vi "ConvertTextBasedCodeToLabVIEW_FixIndexer.vi"(11 "IndexerTextIn":string) -> (3 "MofifiedIndexerTextOut":string)   [LabVIEW 2020]
uses:
  <vilib>/regexp/Match Regular Expression.xnode
panel:
  out "AfterIndexCode 2":string
  out "BeforeIndexCode":string
  out "substring":string
  out "BlockText":string
  out "whole match":string
  # "public string this[int i]\n       {\n          get { return arr[i]; }\n          set { arr[i] = value; }\n       }"
  # "public T this[int i] => arr[i];"
  # "string this[int index]\n    {\n        get;\n        set;\n    }"
  # "string ICitizen.this[int index]\n{\n}"
  # "public T this[int i]\n   {\n      get => arr[i];\n      set => arr[i] = value;\n   }"
  # "string IEmployee.this[int index]\n{\n}"
  # "string IIndexInterface.this[int index]\n{\n}"
  # "public int this[int i]\n    {\n        get { return _values[i]; }\n        set { _values[i] = value; }\n    }"
  # "public int this[int i]\n    {\n        get => _values[i];\n        set => _values[i] = value;\n    }"
  # "public object this[string name]\n        {\n            get => ConfigurationManager.getProperty(name);\n            set => ConfigurationManager.editProperty(name, value);\n        }"
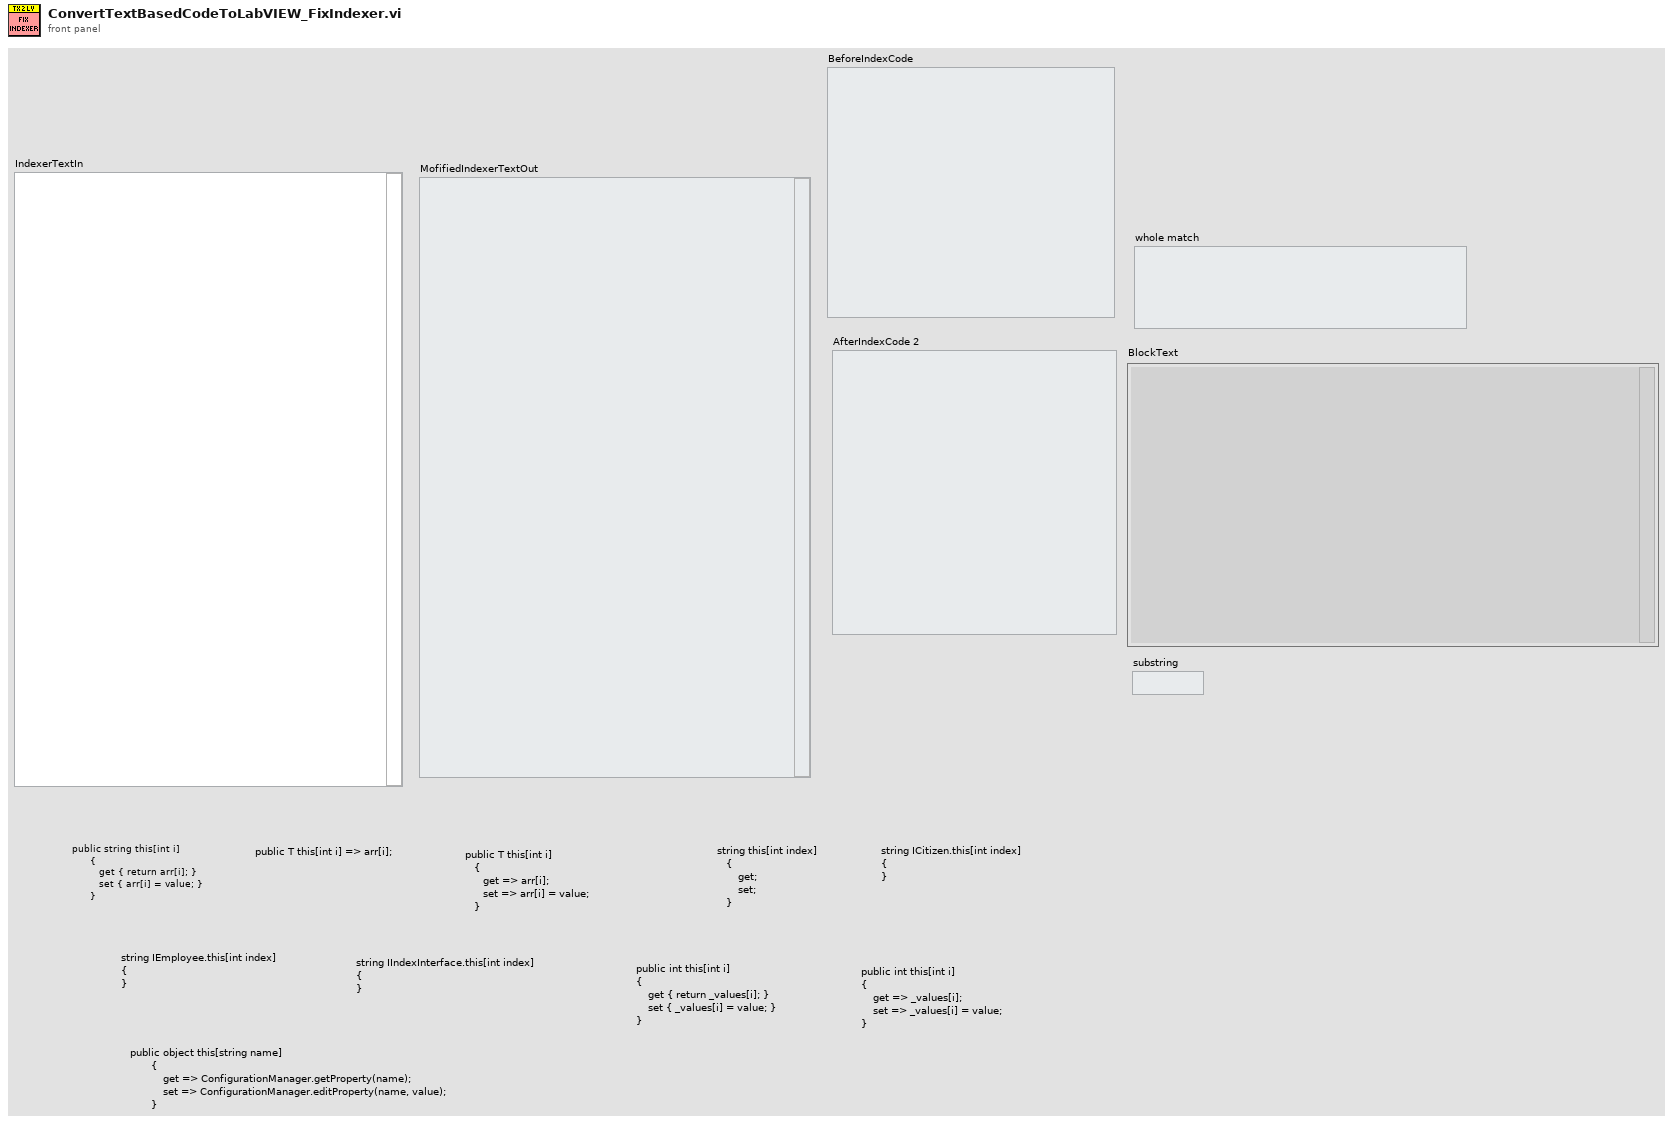
[diagram p1: front panel]
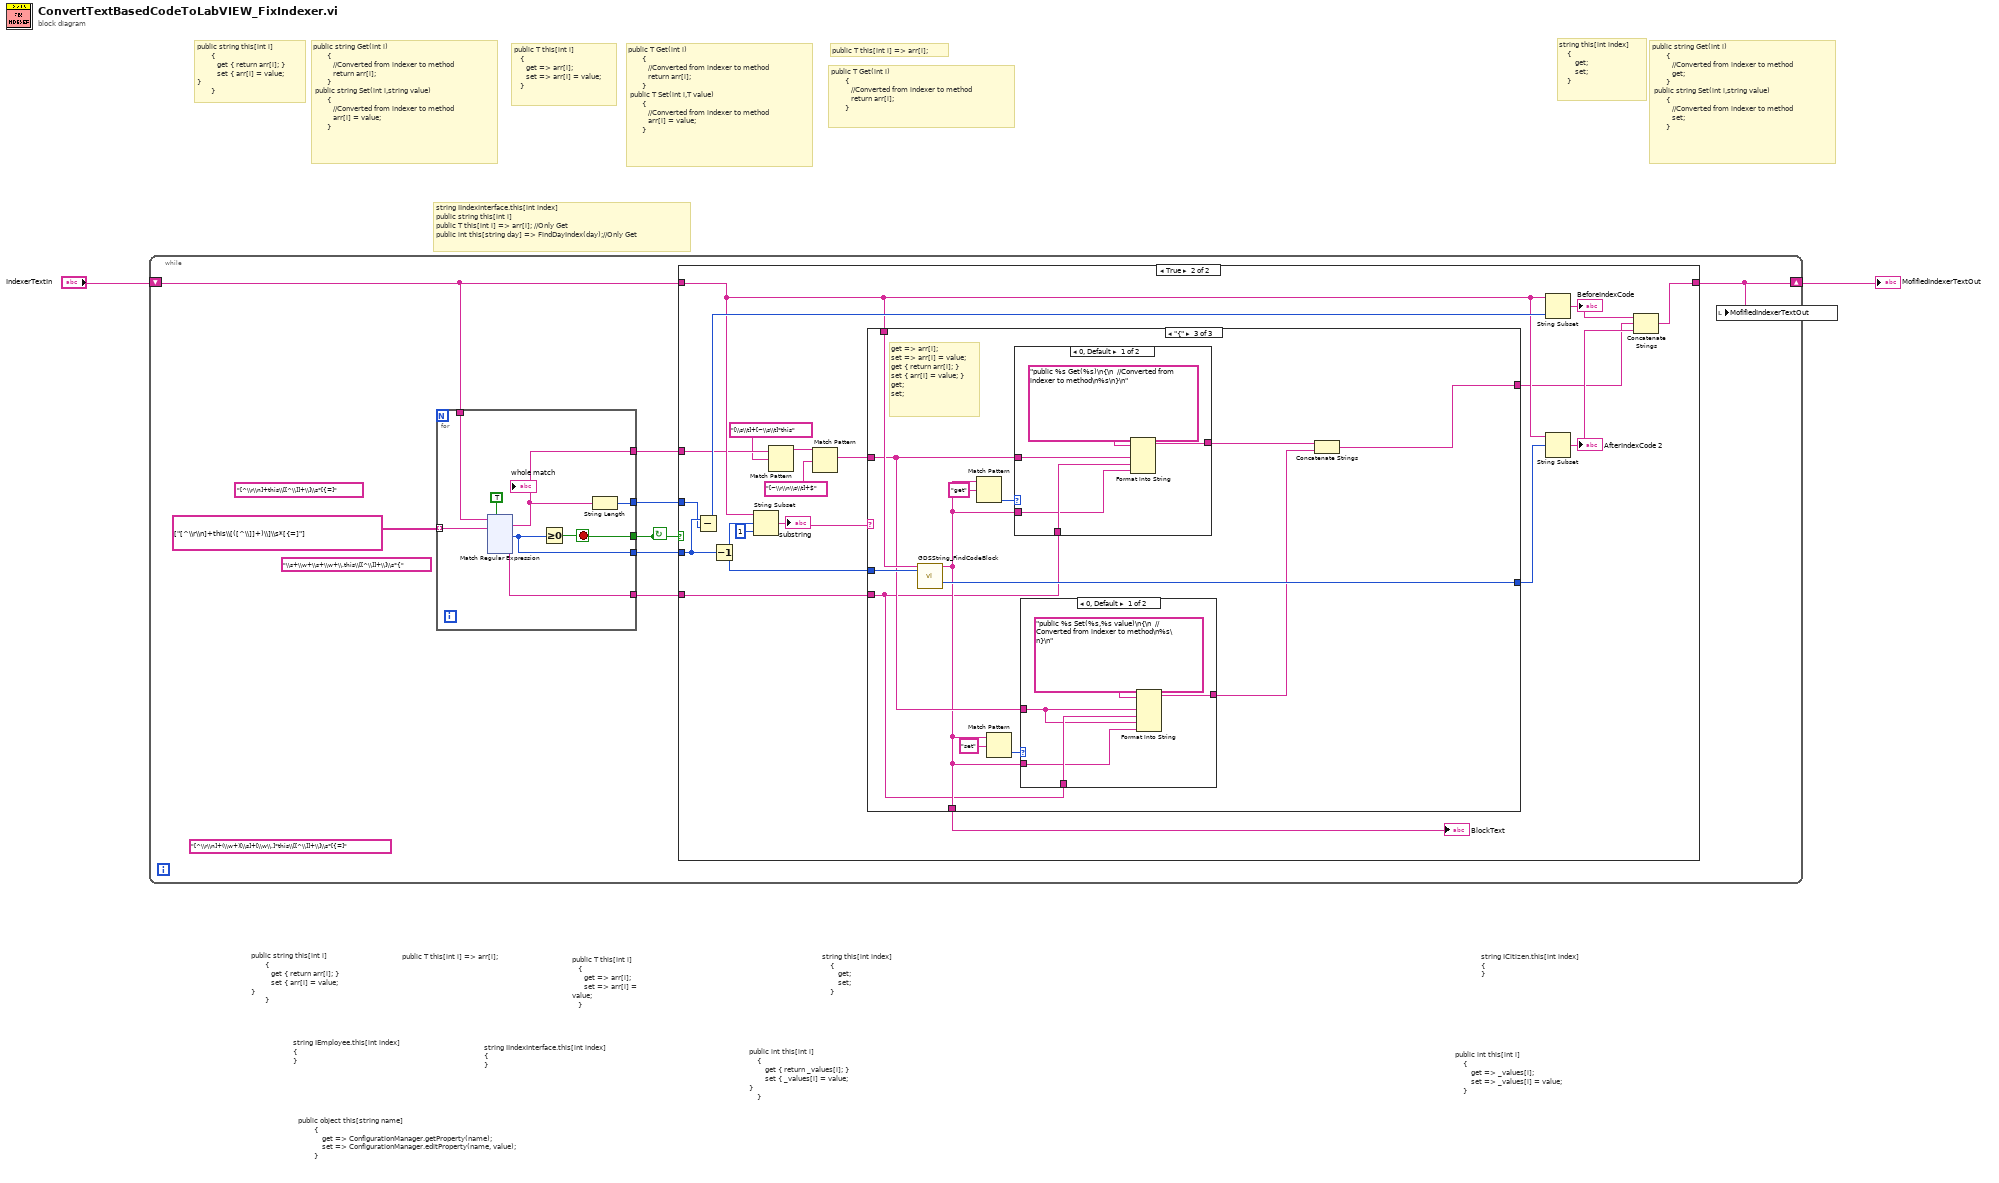
[diagram p0: block diagram]
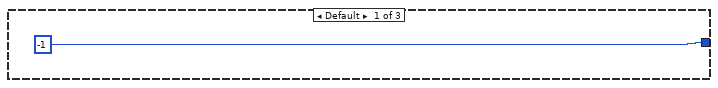
[diagram p3: hidden frame]
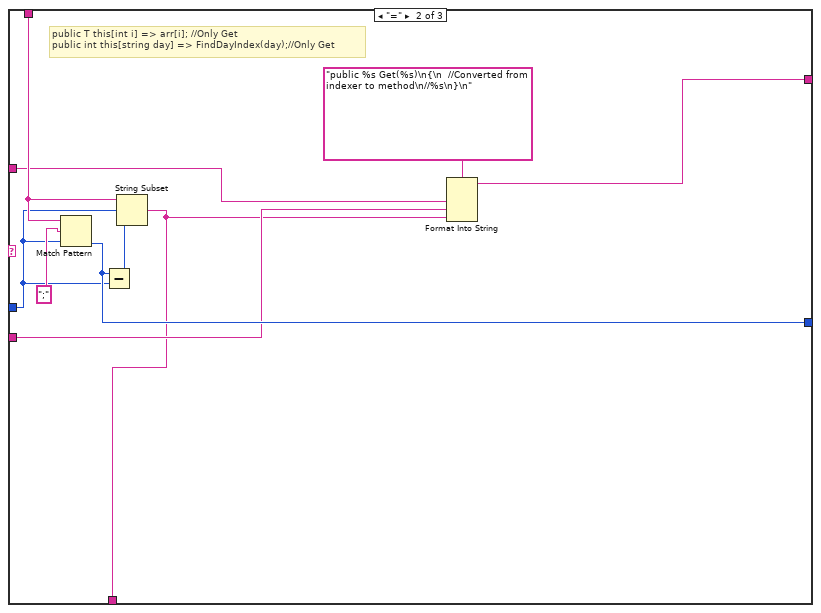
[diagram p4: hidden frame]
diagram:
  # "public string Get(int i)\n       {\n          //Converted from indexer to method\n          get;\n       }\n public string Set(int i,string value)\n       {\n          //Converted from indexer to method\n          set;\n       }"
  # "string this[int index]\n    {\n        get;\n        set;\n    }"
  # "public T Get(int i)\n       {\n          //Converted from indexer to method\n          return arr[i];\n       }"
  # "public T this[int i] => arr[i];"
  # "public T Get(int i)\n       {\n          //Converted from indexer to method\n          return arr[i];\n       }\n public T Set(int i,T value)\n       {\n          //Converted from indexer to method\n          arr[i] = value;\n       }"
  # "public T this[int i]\n   {\n      get => arr[i];\n      set => arr[i] = value;\n   }"
  # "public string Get(int i)\n       {\n          //Converted from indexer to method\n          return arr[i];\n       }\n public string Set(int i,string value)\n       {\n          //Converted from indexer to method\n          arr[i] = value;\n       }"
  # "public string this[int i]\n       {\n          get { return arr[i]; }\n          set { arr[i] = value; }\n       }"
  # "string IIndexInterface.this[int index]\npublic string this[int i]\npublic T this[int i] => arr[i]; //Only Get\npublic int this[string day] => FindDayIndex(day);//Only Get"
  # "public object this[string name]\n        {\n            get => ConfigurationManager.getProperty(name);\n            set => ConfigurationManager.editProperty(name, value);\n        }"
  # "public int this[int i]\n    {\n        get => _values[i];\n        set => _values[i] = value;\n    }"
  # "public int this[int i]\n    {\n        get { return _values[i]; }\n        set { _values[i] = value; }\n    }"
  # "string IIndexInterface.this[int index]\n{\n}"
  # "string IEmployee.this[int index]\n{\n}"
  # "string ICitizen.this[int index]\n{\n}"
  # "string this[int index]\n    {\n        get;\n        set;\n    }"
  # "public T this[int i]\n   {\n      get => arr[i];\n      set => arr[i] = value;\n   }"
  # "public T this[int i] => arr[i];"
  # "public string this[int i]\n       {\n          get { return arr[i]; }\n          set { arr[i] = value; }\n       }"
  n1 = while {
    shift-right: [w5] -> w1
    shift-left: "IndexerTextIn" -> [w8]
    stop <- w7 continue-if-true
    (unwired) "[^\\r\\n]+(\\w+)[\\s]+[\\w\\.]*this\\[[^\\]]+\\]\\s*[{=]" ("input string")
    (unwired) "[^\\r\\n]+this\\[[^\\]]+\\]\\s*[{=]" ("input string")
    (unwired) "\\s+\\w+\\s+\\w+\\.this\\[[^\\]]+\\]\\s*{" ("input string")
    n2 = for {
      tunnel: string[] ["[^\\r\\n]+this\\[([^\\]]+)\\]\\s*[{=]"] ("input string") -> [w71] mode=indexing
      tunnel: w8 -> [w70]
      tunnel: [w69] -> w9
      tunnel: [w68] -> w7
      tunnel: [w67] -> w6
      tunnel: [w66] -> w4
      tunnel: [w65] -> w3
      stop <- w68 stop-if-true
      n3 = xnode "Match Regular Expression"("input string"=w70, "regular expression"=w71, "ignore case? (F)"=TRUE) -> ("whole match"=w66:string, "offset past match"=w69:i32, "submatch 1"=w65:string)  [unwired: 3 in, 3 out]
      "whole match" <- w66
      n4 = Greater Or Equal To 0?(x=w69) -> (x >= 0?=w68:bool)
      n5 = String Length(string=w66) -> (length=w67:i32)
    }
    n6 = case shown="True" w7 {
      tunnel: w9 -> [_ w26]
      tunnel: w8 -> [w11 w20]
      tunnel: [w11 w21] -> w5
      tunnel: w6 -> [_ w25]
      tunnel: w4 -> [_ w18]
      tunnel: w3 -> [_ w13]
      frame False {
      }
      frame True {
        n7 = Subtract(x=w26, y=w25) -> (x-y=w24:i32)
        n8 = Decrement(x=w26) -> (x-1=w30:i32)
        n9 = String Subset(string=w20, offset (0)=w30, length (rest)=1 ("length (rest)")) -> (substring=w28:string)
        "substring" <- w28
        n10 = Match Pattern(string=w18, regular expression="[\\s\\t]+[~\\s\\t]*this") -> (before substring=w16:string)  [unwired: 1 in, 3 out]
        n11 = Match Pattern(string=w16, regular expression="[~\\r\\n\\s\\t]+$") -> (match substring=w14:string)  [unwired: 1 in, 3 out]
        n12 = case shown="\"{\"" w28 {
          tunnel: [_ w33 w46] -> w27
          tunnel: w30 -> [_ w38 w54]
          tunnel: w20 -> [_ w40 w53]
          tunnel: [-1 ("BlockEnd(Outside)") w39 w52] -> w23
          tunnel: w14 -> [_ w36 w47]
          tunnel: w13 -> [_ w34 w45]
          tunnel: [_ w32 w42] -> w12
          frame Default {
          }
          frame "=" {
            # "public T this[int i] => arr[i]; //Only Get\npublic int this[string day] => FindDayIndex(day);//Only Get"
            n13 = Match Pattern(string=w40, regular expression=";", offset (0)=w38) -> (offset past match=w39:i32)  [unwired: 3 out]
            n14 = Subtract(x=w39, y=w38) -> (x-y=w37:i32)
            n15 = String Subset(string=w40, offset (0)=w38, length (rest)=w37) -> (substring=w33:string)
            n16 = Format Into String(format string="public %s Get(%s)\n{\n  //Converted from indexer to method\n//%s\n}\n", w36, w34, w33) -> (resulting string=w32:string)  [unwired: 2 in, 1 out]
          }
          frame "{" {
            # "get => arr[i];\nset => arr[i] = value;\nget { return arr[i]; }\nset { arr[i] = value; }\nget;\nset;"
            n17 = call <resource>:"GDSString_FindCodeBlock.vi"("Text"=w53, "StringStartOffset(Default=-1 => 0 for Forward, StrLenght for Backwards)"=w54) -> ("BlockText"=w46:string, "BlockEnd(Outside)"=w52:i32)  [unwired: 9 in, 7 out]
            n18 = Match Pattern(string=w46, regular expression="get") -> (offset past match=w50:i32)  [unwired: 1 in, 3 out]
            n19 = Match Pattern(string=w46, regular expression="set") -> (offset past match=w48:i32)  [unwired: 1 in, 3 out]
            n20 = case shown="0, Default" w50 {
              tunnel: w47 -> [w63 _]
              tunnel: w45 -> [w62 _]
              tunnel: w46 -> [w61 _]
              tunnel: [w60 _] -> w44
              frame 0, Default {
                n21 = Format Into String(format string="public %s Get(%s)\n{\n  //Converted from indexer to method\n%s\n}\n", w63, w62, w61) -> (resulting string=w60:string)  [unwired: 2 in, 1 out]
              }
              frame -1 {
              }
            }
            n22 = case shown="0, Default" w48 {
              tunnel: w47 -> [w55 _]
              tunnel: w45 -> [w58 _]
              tunnel: w46 -> [w56 _]
              tunnel: [w57 _] -> w43
              frame 0, Default {
                n23 = Format Into String(format string="public %s Set(%s,%s value)\n{\n  //Converted from indexer to method\n%s\n}\n", w55, w58, w55, w56) -> (resulting string=w57:string)  [unwired: 2 in, 1 out]
              }
              frame -1 {
              }
            }
            n24 = Concatenate Strings(w44, w43) -> (w42:string)
          }
        }
        "BlockText" <- w27
        n25 = String Subset(string=w20, length (rest)=w24) -> (substring=w19:string)  [unwired: 1 in]
        "BeforeIndexCode" <- w19
        n26 = String Subset(string=w20, offset (0)=w23) -> (substring=w22:string)  [unwired: 1 in]
        "AfterIndexCode 2" <- w22
        n27 = Concatenate Strings(w19, w12, w22) -> (w21:string)
      }
    }
    n28 = local write "MofifiedIndexerTextOut"(w5) -> ()
  }
  "MofifiedIndexerTextOut" <- w1
